vi "Reset Lateral Waveform.vi"(8 "error in (no error)":errorcluster, 11 "Model in":refnum<class "Model.lvclass">) -> (0 "error out":errorcluster, 3 "Model out":refnum<class "Model.lvclass">)   [LabVIEW 2015, in "Model.lvclass"]
uses:
  Model.lvclass
  Waveforms/Waveform Factory/Waveform Factory.lvclass
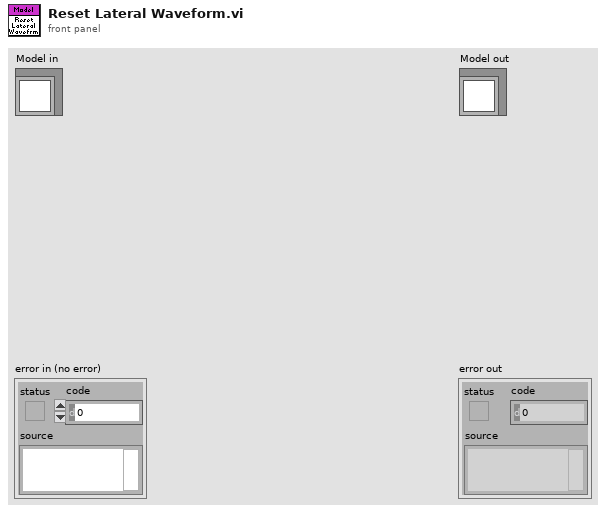
[diagram p1: front panel]
types:
  T1 = typedef "FAMT Typedefs.lvlib/Waveform Settings.ctl" = cluster{"Sample Count":u32, "Amplitude":dbl, "Offset":dbl, "Frequency":dbl[unit], "Waveform":T2, "F1":dbl[unit], "F2":dbl[unit], "Duty Cycle":dbl, "ILC Rate":dbl[unit], "Ramp Time":dbl[unit], "Hold Time":dbl[unit], "Settling Time":dbl[unit], "Delay":dbl[unit]}
  T2 = typedef "FAMT Typedefs.lvlib/Waveform Types.ctl" = enum16{"Sine", "Triangle", "Square", "Sawtooth", "Chirp", "Gaussian", "Trapezoid"}
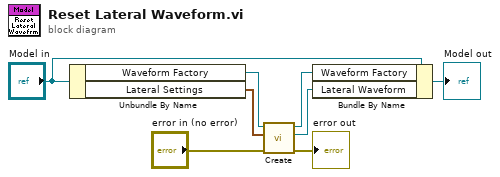
[diagram p0: block diagram]
diagram:
  n1 = Unbundle By Name("Model in") -> ("Waveform Factory"=w6:refnum<class "Waveform Factory.lvclass">, "Lateral Settings"=w5:T1)
  n2 = call-dynamic "Create.vi"("error in (no error)"="error in (no error)", "Waveform Settings"=w5, "Waveform Factory in"=w6) -> ("error out"=→"error out":errorcluster, "Waveform"=w2:refnum<class "Waveform.lvclass">, "Waveform Factory out"=w1:refnum<class "Waveform Factory.lvclass">)  [unwired: 6 in]
  n3 = Bundle By Name(cluster="Model in", "Waveform Factory"=w1, "Lateral Waveform"=w2) -> (→"Model out":refnum<class "Model.lvclass">)
